vi "高精度写.vi"(0 "电压幅值":sgl, 1 "电压纹波":sgl, 2 "串口号":refnum<visa-resource-name>, 5 "电压档位":u32, 7 "电流幅值":sgl, 9 "电流档位值":u32, 11 "纹波频率":sgl, 12 "电流纹波":sgl, 14 "电流通道":dbl) -> (8 "应答":string)   [LabVIEW 2014]
panel:
  in  "电流纹波通道":u32
  in  "电流波形类型":sgl
  in  "电流相位通道":sgl
  in  "电流幅值通道":sgl
  in  "电流档位通道":u32
  out "字符串":string
  out "I直流":bool
  out "U直流":bool
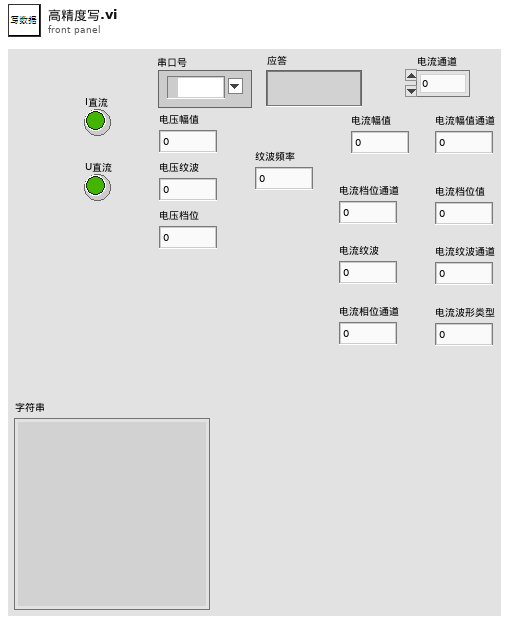
[diagram p1: front panel]
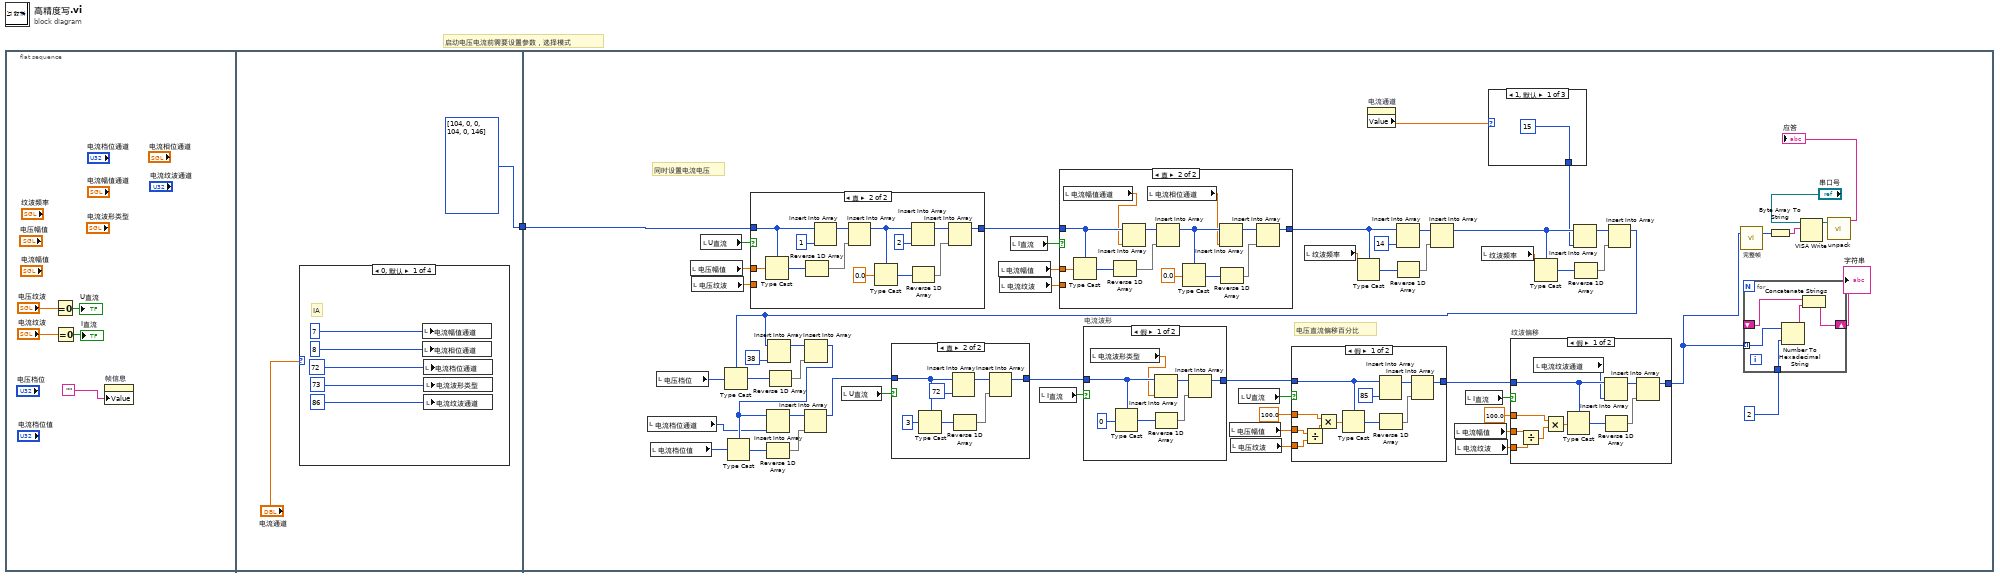
[diagram p0: block diagram]
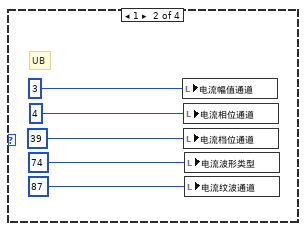
[diagram p2: hidden frame]
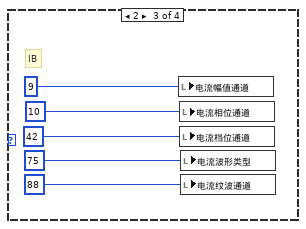
[diagram p3: hidden frame]
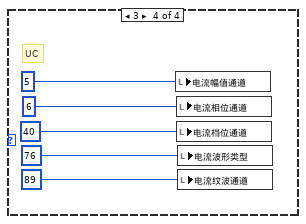
[diagram p4: hidden frame]
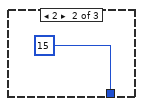
[diagram p5: hidden frame]
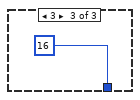
[diagram p6: hidden frame]
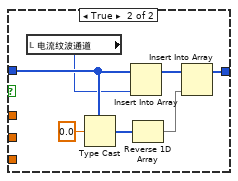
[diagram p7: hidden frame]
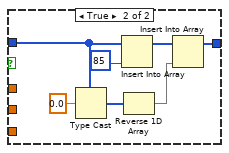
[diagram p8: hidden frame]
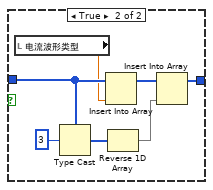
[diagram p9: hidden frame]
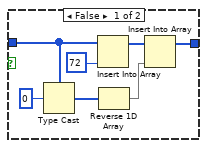
[diagram p10: hidden frame]
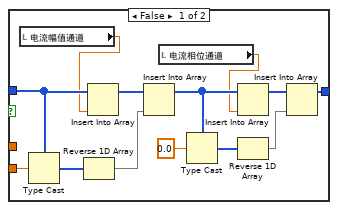
[diagram p11: hidden frame]
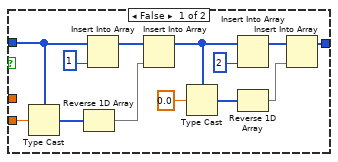
[diagram p12: hidden frame]
diagram:
  # "启动电压电流前需要设置参数，选择模式"
  n1 = flat-sequence {
    tunnel: [u8[] [104, 0, 0, 104, 0, 146]] -> w1
    tunnel: w1 -> [w83]
    frame #0 {
      n2 = Equal To 0?(x="电压纹波") -> (x = 0?=→"U直流":bool)
      n3 = Equal To 0?(x="电流纹波") -> (x = 0?=→"I直流":bool)
      n4 = property on="帧信息" class="Str"("Value"="") -> ()  [unwired: 2 in, 2 out]
    }
    frame #1 {
      n5 = case shown="0, 默认" "电流通道" {
        frame 0, Default {
          # "IA"
          n6 = local write "电流幅值通道"(7) -> ()
          n7 = local write "电流相位通道"(8) -> ()
          n8 = local write "电流档位通道"(72) -> ()
          n9 = local write "电流波形类型"(73) -> ()
          n10 = local write "电流纹波通道"(86) -> ()
        }
        frame 1 {
          # "UB"
          n11 = local write "电流幅值通道"(3) -> ()
          n12 = local write "电流相位通道"(4) -> ()
          n13 = local write "电流档位通道"(39) -> ()
          n14 = local write "电流波形类型"(74) -> ()
          n15 = local write "电流纹波通道"(87) -> ()
        }
        frame 2 {
          # "IB"
          n16 = local write "电流幅值通道"(9) -> ()
          n17 = local write "电流相位通道"(10) -> ()
          n18 = local write "电流档位通道"(42) -> ()
          n19 = local write "电流波形类型"(75) -> ()
          n20 = local write "电流纹波通道"(88) -> ()
        }
        frame 3 {
          # "UC"
          n21 = local write "电流幅值通道"(5) -> ()
          n22 = local write "电流相位通道"(6) -> ()
          n23 = local write "电流档位通道"(40) -> ()
          n24 = local write "电流波形类型"(76) -> ()
          n25 = local write "电流纹波通道"(89) -> ()
        }
      }
    }
    frame #2 {
      # "电压直流偏移百分比"
      # "同时设置电流电压"
      n26 = local read "电流档位通道"() -> (w42:u32)
      n27 = local read "电流档位值"() -> (w43:u32)
      n28 = local read "电压档位"() -> (w44:u32)
      n29 = local read "电压幅值"() -> (w78:sgl)
      n30 = local read "电压纹波"() -> (w77:sgl)
      n31 = local read "U直流"() -> (w79:bool)
      n32 = case shown="真" w79 {
        tunnel: w83 -> [w183 w203]
        tunnel: [w184 w196] -> w73
        tunnel: w78 -> [_ w195]
        tunnel: w77 -> [w182 _]
        frame False {
          n33 = Type Cast(type=w183, x=w182) -> (*(type *) &x=w193:u8[])
          n34 = Reverse 1D Array(array=w193) -> (reversed array=w194:u8[])
          n35 = Insert Into Array(array=w183, new element=u8 1 ("新元素/子数组")) -> (w192:u8[])  [unwired: 1 in]
          n36 = Insert Into Array(array=w192, new element=w194) -> (w185:u8[])  [unwired: 1 in]
          n37 = Type Cast(type=w185, x=sgl 0.0) -> (*(type *) &x=w188:u8[])
          n38 = Insert Into Array(array=w185, new element=u8 2 ("新元素/子数组")) -> (w186:u8[])  [unwired: 1 in]
          n39 = Reverse 1D Array(array=w188) -> (reversed array=w190:u8[])
          n40 = Insert Into Array(array=w186, new element=w190) -> (w184:u8[])  [unwired: 1 in]
        }
        frame True {
          n41 = Type Cast(type=w203, x=w195) -> (*(type *) &x=w206:u8[])
          n42 = Reverse 1D Array(array=w206) -> (reversed array=w207:u8[])
          n43 = Insert Into Array(array=w203, new element=u8 1 ("新元素/子数组")) -> (w205:u8[])  [unwired: 1 in]
          n44 = Insert Into Array(array=w205, new element=w207) -> (w197:u8[])  [unwired: 1 in]
          n45 = Type Cast(type=w197, x=sgl 0.0) -> (*(type *) &x=w200:u8[])
          n46 = Insert Into Array(array=w197, new element=u8 2 ("新元素/子数组")) -> (w198:u8[])  [unwired: 1 in]
          n47 = Reverse 1D Array(array=w200) -> (reversed array=w202:u8[])
          n48 = Insert Into Array(array=w198, new element=w202) -> (w196:u8[])  [unwired: 1 in]
        }
      }
      n49 = local read "U直流"() -> (w63:bool)
      n50 = local read "电流幅值"() -> (w75:sgl)
      n51 = local read "电流纹波"() -> (w76:sgl)
      n52 = local read "I直流"() -> (w74:bool)
      n53 = local read "I直流"() -> (w62:bool)
      n54 = case shown="真" w74 {
        tunnel: w73 -> [w159 w178]
        tunnel: [w160 w172] -> w72
        tunnel: w75 -> [_ w171]
        tunnel: w76 -> [w158 _]
        frame False {
          n55 = local read "电流幅值通道"() -> (w157:sgl)
          n56 = Type Cast(type=w159, x=w158) -> (*(type *) &x=w167:u8[])
          n57 = Reverse 1D Array(array=w167) -> (reversed array=w168:u8[])
          n58 = Insert Into Array(array=w159, new element=w157) -> (w166:u8[])  [unwired: 1 in]
          n59 = Insert Into Array(array=w166, new element=w168) -> (w161:u8[])  [unwired: 1 in]
          n60 = local read "电流相位通道"() -> (w156:sgl)
          n61 = Type Cast(type=w161, x=sgl 0.0) -> (*(type *) &x=w163:u8[])
          n62 = Insert Into Array(array=w161, new element=w156) -> (w162:u8[])  [unwired: 1 in]
          n63 = Reverse 1D Array(array=w163) -> (reversed array=w165:u8[])
          n64 = Insert Into Array(array=w162, new element=w165) -> (w160:u8[])  [unwired: 1 in]
        }
        frame True {
          n65 = local read "电流幅值通道"() -> (w170:sgl)
          n66 = Type Cast(type=w178, x=w171) -> (*(type *) &x=w180:u8[])
          n67 = Reverse 1D Array(array=w180) -> (reversed array=w181:u8[])
          n68 = Insert Into Array(array=w178, new element=w170) -> (w179:u8[])  [unwired: 1 in]
          n69 = local read "电流相位通道"() -> (w169:sgl)
          n70 = Insert Into Array(array=w179, new element=w181) -> (w173:u8[])  [unwired: 1 in]
          n71 = Type Cast(type=w173, x=sgl 0.0) -> (*(type *) &x=w175:u8[])
          n72 = Insert Into Array(array=w173, new element=w169) -> (w174:u8[])  [unwired: 1 in]
          n73 = Reverse 1D Array(array=w175) -> (reversed array=w177:u8[])
          n74 = Insert Into Array(array=w174, new element=w177) -> (w172:u8[])  [unwired: 1 in]
        }
      }
      n75 = local read "电压幅值"() -> (w57:sgl)
      n76 = local read "电压纹波"() -> (w56:sgl)
      n77 = local read "U直流"() -> (w59:bool)
      n78 = local read "纹波频率"() -> (w41:sgl)
      n79 = Type Cast(type=w72, x=w41) -> (*(type *) &x=w39:u8[])
      n80 = property on="电流通道" class="DigNum (严格)"() -> ("Value"=w36:dbl)  [unwired: 2 in, 2 out]
      n81 = Insert Into Array(array=w72, new element=u8 14 ("新元素/子数组")) -> (w38:u8[])  [unwired: 1 in]
      n82 = Reverse 1D Array(array=w39) -> (reversed array=w40:u8[])
      n83 = Insert Into Array(array=w38, new element=w40) -> (w30:u8[])  [unwired: 1 in]
      n84 = local read "电流幅值"() -> (w54:sgl)
      n85 = local read "电流纹波"() -> (w55:sgl)
      n86 = local read "I直流"() -> (w53:bool)
      n87 = local read "纹波频率"() -> (w32:sgl)
      n88 = case shown="1, 默认" w36 {
        tunnel: [15 15 16] -> w29
        frame 1, Default {
        }
        frame 2 {
        }
        frame 3 {
        }
      }
      n89 = Type Cast(type=w30, x=w32) -> (*(type *) &x=w34:u8[])
      n90 = Insert Into Array(array=w30, new element=w29) -> (w35:u8[])  [unwired: 1 in]
      n91 = Reverse 1D Array(array=w34) -> (reversed array=w33:u8[])
      n92 = Insert Into Array(array=w35, new element=w33) -> (w31:u8[])  [unwired: 1 in]
      n93 = Type Cast(type=w31, x=w44) -> (*(type *) &x=w69:u8[])
      n94 = Insert Into Array(array=w31, new element=u8 38 ("新元素/子数组")) -> (w70:u8[])  [unwired: 1 in]
      n95 = Reverse 1D Array(array=w69) -> (reversed array=w68:u8[])
      n96 = Insert Into Array(array=w70, new element=w68) -> (w64:u8[])  [unwired: 1 in]
      n97 = Type Cast(type=w64, x=w43) -> (*(type *) &x=w66:u8[])
      n98 = Insert Into Array(array=w64, new element=w42) -> (w65:u8[])  [unwired: 1 in]
      n99 = Reverse 1D Array(array=w66) -> (reversed array=w67:u8[])
      n100 = Insert Into Array(array=w65, new element=w67) -> (w61:u8[])  [unwired: 1 in]
      n101 = case shown="真" w63 {
        tunnel: w61 -> [w144 w151]
        tunnel: [w143 w149] -> w60
        frame False {
          n102 = Type Cast(type=w144, x=u32 0) -> (*(type *) &x=w147:u8[])
          n103 = Insert Into Array(array=w144, new element=u8 72 ("新元素/子数组")) -> (w146:u8[])  [unwired: 1 in]
          n104 = Reverse 1D Array(array=w147) -> (reversed array=w148:u8[])
          n105 = Insert Into Array(array=w146, new element=w148) -> (w143:u8[])  [unwired: 1 in]
        }
        frame True {
          n106 = Type Cast(type=w151, x=u32 3) -> (*(type *) &x=w154:u8[])
          n107 = Insert Into Array(array=w151, new element=u8 72 ("新元素/子数组")) -> (w153:u8[])  [unwired: 1 in]
          n108 = Reverse 1D Array(array=w154) -> (reversed array=w155:u8[])
          n109 = Insert Into Array(array=w153, new element=w155) -> (w149:u8[])  [unwired: 1 in]
        }
      }
      n110 = case "电流波形" shown="假" w62 {
        tunnel: w60 -> [w131 w138]
        tunnel: [w130 w137] -> w58
        frame False {
          n111 = local read "电流波形类型"() -> (w128:sgl)
          n112 = Type Cast(type=w131, x=u32 0) -> (*(type *) &x=w133:u8[])
          n113 = Insert Into Array(array=w131, new element=w128) -> (w132:u8[])  [unwired: 1 in]
          n114 = Reverse 1D Array(array=w133) -> (reversed array=w134:u8[])
          n115 = Insert Into Array(array=w132, new element=w134) -> (w130:u8[])  [unwired: 1 in]
        }
        frame True {
          n116 = local read "电流波形类型"() -> (w135:sgl)
          n117 = Type Cast(type=w138, x=u32 3) -> (*(type *) &x=w140:u8[])
          n118 = Insert Into Array(array=w138, new element=w135) -> (w139:u8[])  [unwired: 1 in]
          n119 = Reverse 1D Array(array=w140) -> (reversed array=w141:u8[])
          n120 = Insert Into Array(array=w139, new element=w141) -> (w137:u8[])  [unwired: 1 in]
        }
      }
      n121 = case shown="假" w59 {
        tunnel: w58 -> [w116 w123]
        tunnel: [w115 w122] -> w52
        tunnel: w57 -> [w114 _]
        tunnel: w56 -> [w113 _]
        tunnel: sgl 100.0 ("x") -> [w110 _]
        frame False {
          n122 = Divide(x=w114, y=w113) -> (x/y=w111:sgl)
          n123 = Multiply(x=w110, y=w111) -> (x*y=w112:sgl)
          n124 = Type Cast(type=w116, x=w112) -> (*(type *) &x=w119:u8[])
          n125 = Insert Into Array(array=w116, new element=u8 85 ("新元素/子数组")) -> (w118:u8[])  [unwired: 1 in]
          n126 = Reverse 1D Array(array=w119) -> (reversed array=w120:u8[])
          n127 = Insert Into Array(array=w118, new element=w120) -> (w115:u8[])  [unwired: 1 in]
        }
        frame True {
          n128 = Type Cast(type=w123, x=sgl 0.0) -> (*(type *) &x=w126:u8[])
          n129 = Insert Into Array(array=w123, new element=u8 85 ("新元素/子数组")) -> (w125:u8[])  [unwired: 1 in]
          n130 = Reverse 1D Array(array=w126) -> (reversed array=w127:u8[])
          n131 = Insert Into Array(array=w125, new element=w127) -> (w122:u8[])  [unwired: 1 in]
        }
      }
      n132 = case "纹波偏移" shown="假" w53 {
        tunnel: w52 -> [w99 w106]
        tunnel: [w98 w105] -> w46
        tunnel: w54 -> [w97 _]
        tunnel: w55 -> [w96 _]
        tunnel: sgl 100.0 ("x") -> [w93 _]
        frame False {
          n133 = Divide(x=w97, y=w96) -> (x/y=w94:sgl)
          n134 = local read "电流纹波通道"() -> (w92:u32)
          n135 = Multiply(x=w93, y=w94) -> (x*y=w95:sgl)
          n136 = Type Cast(type=w99, x=w95) -> (*(type *) &x=w101:u8[])
          n137 = Insert Into Array(array=w99, new element=w92) -> (w100:u8[])  [unwired: 1 in]
          n138 = Reverse 1D Array(array=w101) -> (reversed array=w102:u8[])
          n139 = Insert Into Array(array=w100, new element=w102) -> (w98:u8[])  [unwired: 1 in]
        }
        frame True {
          n140 = local read "电流纹波通道"() -> (w103:u32)
          n141 = Type Cast(type=w106, x=sgl 0.0) -> (*(type *) &x=w108:u8[])
          n142 = Insert Into Array(array=w106, new element=w103) -> (w107:u8[])  [unwired: 1 in]
          n143 = Reverse 1D Array(array=w108) -> (reversed array=w109:u8[])
          n144 = Insert Into Array(array=w107, new element=w109) -> (w105:u8[])  [unwired: 1 in]
        }
      }
      n145 = call "完整帧.vi"("不完整帧"=w46) -> ("完整帧"=w49:u8[])  [unwired: 2 in]
      n146 = for {
        shift-right: [w90] -> w80
        shift-left: _ -> [w91]
        tunnel: w46 -> [w88] mode=indexing
        tunnel: 2 -> [w87]
        n147 = Number To Hexadecimal String(1:w87, 2:w88) -> (0:w89:string)
        n148 = Concatenate Strings(w91, w89) -> (w90:string)
      }
      "字符串" <- w80
      n149 = Byte Array To String(unsigned byte array=w49) -> (string=w47:string)
      n150 = VISA Write(VISA resource name="串口号", write buffer=w47) -> (VISA resource name out=w48:refnum<visa-resource-name>)  [unwired: 1 in, 2 out]
      n151 = call "unpack.vi"("串口号输入"=w48) -> ("应答"=→"应答":string)  [unwired: 5 in, 1 out]
    }
  }
